vi "RemoveExternalDependencies.vi"(8 "error in (no error)":errorcluster, 9 "Possible deps":set{string}(c389), 11 "ProjectItem in":refnum<class "ProjectItem.lvclass">) -> (0 "error out":errorcluster, 3 "ProjectItem out":refnum<class "ProjectItem.lvclass">)   [LabVIEW 2019, in "SolutionBuilder.lvlib" / "ProjectItem.lvclass"]
uses:
  ProjectItem.lvclass
  ProjectItem.lvclass/ProjectItem.ctl
  4de0adc9-0dd1-42b8-8cf9-69e6116373ab.vi
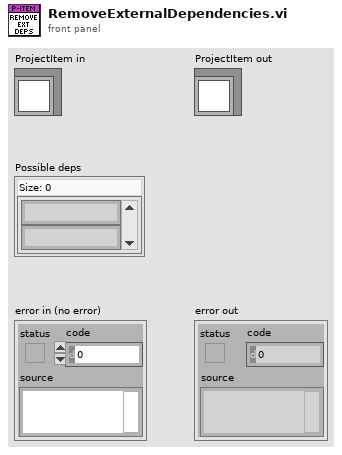
[diagram p1: front panel]
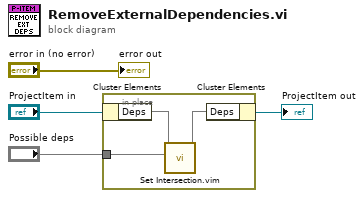
[diagram p0: block diagram]
diagram:
  n1 = in-place {
    in-place-border: "Possible deps" -> [w6]
    n2 = in-place-cluster #1("ProjectItem in") -> ("Deps"=w7:set{string})
    n3 = call "Set Intersection.vim"("set 2"=w6, "set 1"=w7) -> ("intersection"=w5:set{string})  [unwired: 9 in]
    n4 = in-place-cluster #1("Deps"=w5) -> (→"ProjectItem out":refnum<class "ProjectItem.lvclass">)
  }
  "error out" <- "error in (no error)"
